vi "RPi WebDAV.vi"(8 "Error IN":errorcluster, 9 "RPi Sub-Dir":string="Sync", 10 "RPi IP":string="10.31.176.22", 11 "RIO Folder":path=path "c:/Closed_Data") -> (0 "Error OUT":errorcluster, 3 "Files Paths":path[](array[path]))   [LabVIEW 2013]
uses:
  <vilib>/WebDAVClient/Advanced/Put File.vi
  <vilib>/WebDAVClient/NI_WebDAV.lvlib
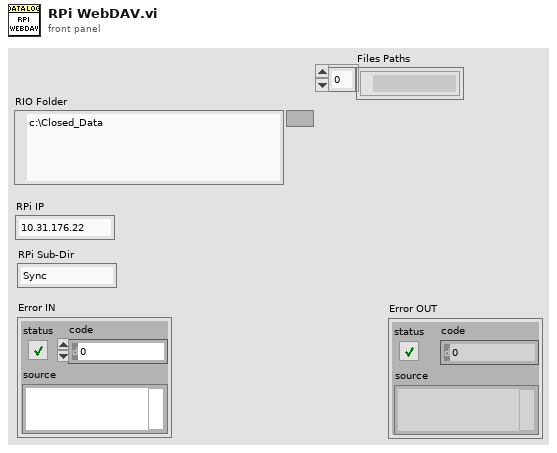
[diagram p1: front panel]
types:
  T1 = typedef "NI_WebDAV.lvlib/SessionHandle.ctl" = refnum<k1>
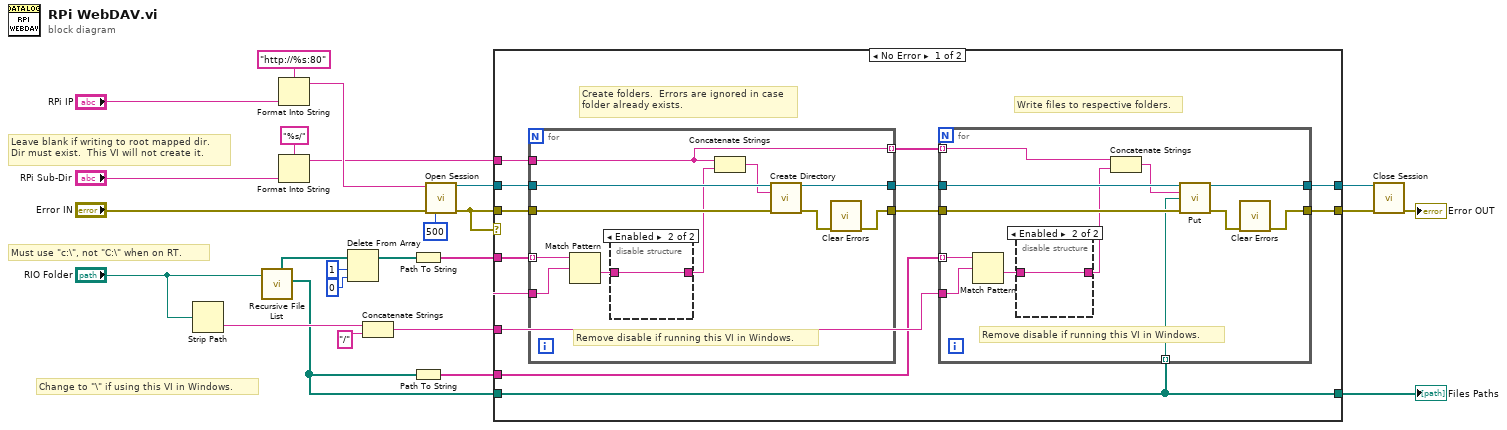
[diagram p0: block diagram]
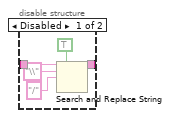
[diagram p2: hidden frame]
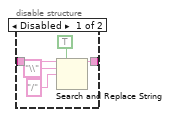
[diagram p3: hidden frame]
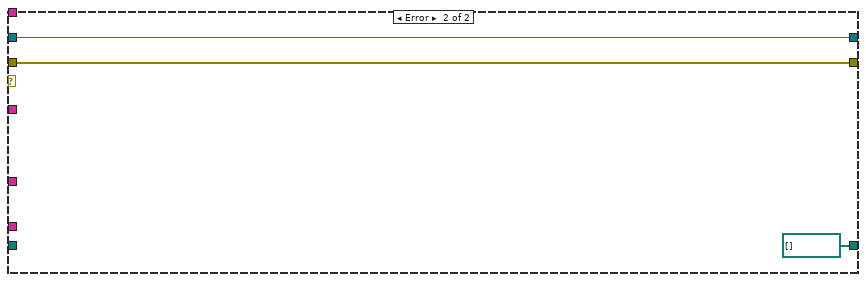
[diagram p4: hidden frame]
diagram:
  # "Leave blank if writing to root mapped dir.\nDir must exist.  This VI will not create it."
  # "Change to \"\\\" if using this VI in Windows."
  # "Must use \"c:\\\", not \"C:\\\" when on RT."
  n1 = Strip Path(path="RIO Folder") -> (name=w20:string)  [unwired: 1 out]
  n2 = call <vilib>:"Recursive File List.vi"("Folder Path"="RIO Folder") -> ("All Files in Dir"=w18:path[], "All Folders"=w25:path[])  [unwired: 6 in, 3 out]
  n3 = Format Into String(format string="http://%s:80" ("file uri"), "RPi IP") -> (resulting string=w13:string)  [unwired: 2 in, 1 out]
  n4 = Format Into String(format string="%s/" ("file uri"), "RPi Sub-Dir") -> (resulting string=w4:string)  [unwired: 2 in, 1 out]
  n5 = Delete From Array(array=w25, length=1, index=0) -> (array with subset deleted=w22:path[])  [unwired: 1 out]
  n6 = Concatenate Strings(w20, "/" ("format string")) -> (w19:string)
  n7 = Path To String(path=w22) -> (string=w11:string[])
  n8 = Path To String(path=w18) -> (string=w10:string[])
  n9 = call <vilib>:"Open Session.vi"("host uri prefix"=w13, "error in (no error)"="Error IN", "timeout ms"=500) -> ("session handle out"=w12:T1, "error out"=w3:errorcluster)  [unwired: 11 in]
  n10 = case shown="No Error" w3 {
    tunnel: w19 -> [w37 _]
    tunnel: w18 -> [w26 _]
    tunnel: w3 -> [w36 w75]
    tunnel: w12 -> [w35 w74]
    tunnel: w11 -> [w34 _]
    tunnel: w10 -> [w31 _]
    tunnel: [w30 w74] -> w9
    tunnel: [w29 w75] -> w8
    tunnel: w4 -> [w28 _]
    tunnel: [w26 path[] [] ("All Files in Dir")] -> w1
    frame No Error {
      # "Write files to respective folders."
      # "Create folders.  Errors are ignored in case\nfolder already exists."
      n11 = for {
        tunnel: w36 -> [w65]
        tunnel: w35 -> [w64]
        tunnel: [w63] -> w33
        tunnel: [w62] -> w32
        tunnel: w34 -> [w61] mode=indexing
        tunnel: w37 -> [w60]
        tunnel: w28 -> [w56]
        tunnel: [w56] -> w27 mode=indexing
        # "Remove disable if running this VI in Windows."
        n12 = Match Pattern(string=w61, regular expression=w60) -> (after substring=w59:string)  [unwired: 1 in, 3 out]
        n13 = disable-structure shown="Enabled" {
          disable-tunnel: [w71 w72] -> w58
          disable-tunnel: w59 -> [w69 w72]
          frame Disabled {
            n14 = Search and Replace String(replace all?=TRUE ("replace all? (F)"), input string=w69, search string="\\", replace string="/" ("replace string (\"\")")) -> (result string=w71:string)  [unwired: 4 in, 3 out]
          }
          frame Enabled {
          }
        }
        n15 = Concatenate Strings(w56, w58) -> (w57:string)
        n16 = call <vilib>:"Create Directory.vi"("session handle"=w64, "relative uri"=w57, "error in (no error)"=w65) -> ("session handle out"=w63:T1, "error out"=w66:errorcluster)  [unwired: 11 in]
        n17 = call <vilib>:"Clear Errors.vi"("error in (no error)"=w66) -> ("error out"=w62:errorcluster)  [unwired: 6 in]
      }
      n18 = for {
        tunnel: w32 -> [w48]
        tunnel: w33 -> [w47]
        tunnel: [w46] -> w30
        tunnel: [w45] -> w29
        tunnel: w31 -> [w44] mode=indexing
        tunnel: w37 -> [w43]
        tunnel: w26 -> [w42] mode=indexing
        tunnel: w27 -> [w40] mode=indexing
        # "Remove disable if running this VI in Windows."
        n19 = Match Pattern(string=w44, regular expression=w43) -> (after substring=w41:string)  [unwired: 1 in, 3 out]
        n20 = disable-structure shown="Enabled" {
          disable-tunnel: [w54 w55] -> w39
          disable-tunnel: w41 -> [w52 w55]
          frame Disabled {
            n21 = Search and Replace String(replace all?=TRUE ("replace all? (F)"), input string=w52, search string="\\", replace string="/" ("replace string (\"\")")) -> (result string=w54:string)  [unwired: 4 in, 3 out]
          }
          frame Enabled {
          }
        }
        n22 = Concatenate Strings(w40, w39) -> (w38:string)
        n23 = call-poly <vilib>:"Put.vi"("session handle"=w47, "relative uri"=w38, "local file path"=w42, "error in (no error)"=w48) -> ("session handle out"=w46:T1, "error out"=w49:errorcluster)  [unwired: 9 in, 1 out]
        n24 = call <vilib>:"Clear Errors.vi"("error in (no error)"=w49) -> ("error out"=w45:errorcluster)  [unwired: 6 in]
      }
    }
    frame Error {
    }
  }
  "Files Paths" <- w1
  n25 = call <vilib>:"Close Session.vi"("session handle"=w9, "error in (no error)"=w8) -> ("error out"=→"Error OUT":errorcluster)  [unwired: 13 in]
